vi "DataSimulation.vi"(8 "error in (no error)":errorcluster) -> (0 "error out":errorcluster)   [LabVIEW 2020]
uses:
  StateGPSUpdate.ctl
  <vilib>/Skyline/Message/NI Skyline Message.lvclass
  <vilib>/Skyline/Tag/Shared/typedefs/DataType.ctl
  <vilib>/Skyline/Configuration/Configuration HTTP_class/NI Skyline Configuration HTTP.lvclass/NI Skyline Configuration HTTP.ctl
  TestData.ctl
  <vilib>/Skyline/Configuration/Configuration HTTP_class/Open Configuration HTTP.vi
  <vilib>/Skyline/Message/HTTP Wrapper/NI Skyline Message HTTP.lvclass
  C:/Program Files (x86)/National Instruments/LabVIEW 2020/vi.lib/Skyline/Message/NI Skyline Message.lvclass
  <vilib>/Skyline/Configuration/HTTP/Open Configuration (Desktop).vi
  <vilib>/Skyline/Tag/Wrapper/Wrapper HTTP_class/Open Tag HTTP.vi
  <vilib>/Skyline/Tag/Wrapper/Wrapper_class/Write Tag (Timestamp).vi
  <vilib>/Skyline/Message/HTTP Wrapper/Open (HTTP).vi
  <vilib>/Skyline/Tag/Wrapper/Wrapper_class/Write Tag (Boolean).vi
  <vilib>/Skyline/Configuration/Configuration HTTP_class/NI Skyline Configuration HTTP.lvclass
  <vilib>/Skyline/Configuration/Configuration_class/NI Skyline Configuration.lvclass
  <vilib>/Skyline/Utilities/NI Skyline Utilities.lvlib
  <vilib>/Skyline/Tag/Wrapper/Wrapper_class/NI Skyline Tag.lvclass
  <vilib>/Skyline/Tag/Shared/NI Skyline Tag.lvlib
  <vilib>/Skyline/Tag/Wrapper/Wrapper HTTP_class/NI Skyline Tag HTTP.lvclass
panel:
  in  "stop":bool
  out "Connection Status":bool
  out "SystemStartTime":timestamp
  in  "Test Drive Distance":dbl=1000.0
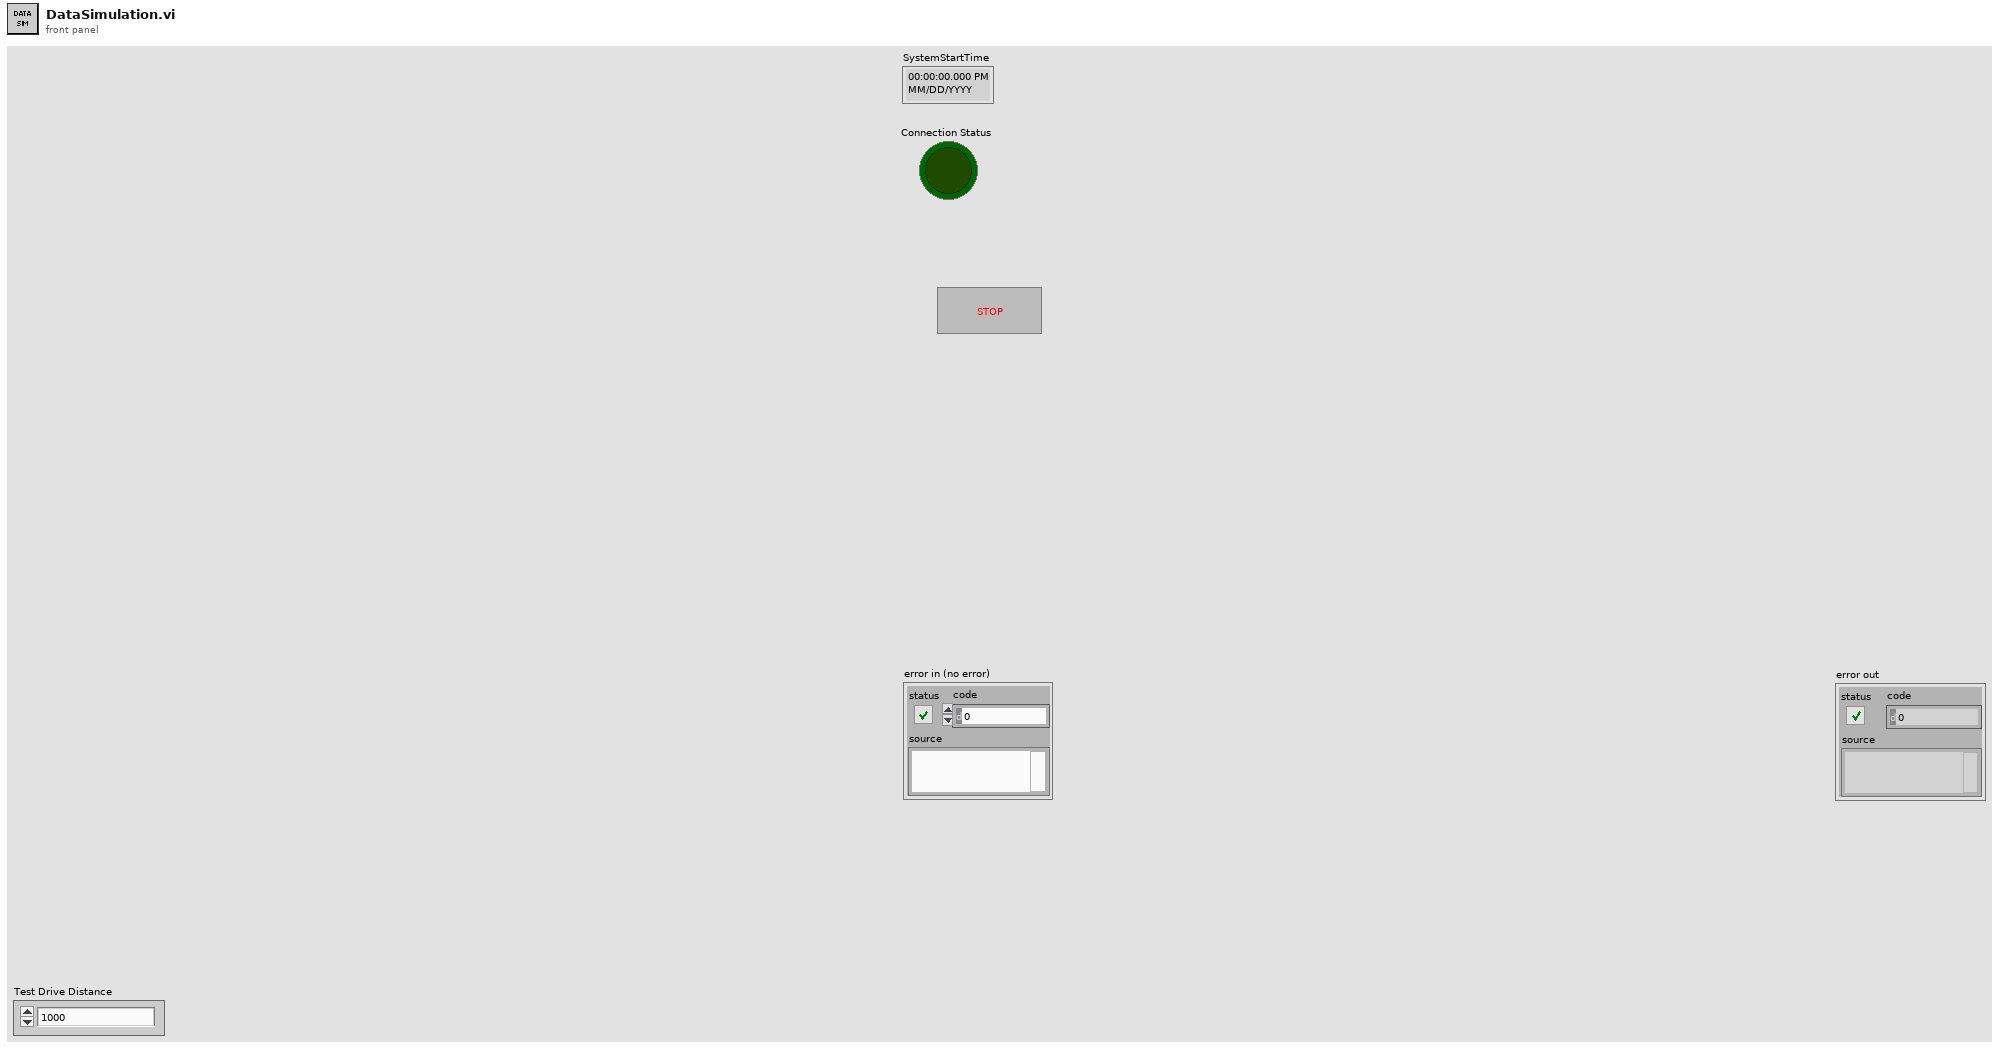
[diagram p1: front panel]
types:
  T1 = typedef "StateGPSUpdate.ctl" = enum16{"Init", "UpdateGPS", "Shutdown"}
  T2 = typedef "NI Skyline Tag.lvlib/DataType.ctl" = enum32{"Double", "I32", "String", "Boolean", "U64", "Timestamp"}
  T3 = typedef "TestData.ctl" = cluster{"GPS":cluster{"Latitude":dbl, "Longitude":dbl, "Timestamp":string}, "SystemLinkClientInfo":cluster{"TargetName":string, "MinionID":string}, "CampaignData":cluster{"DistanceTraveled":dbl, "CampaignProgress":dbl, "Speed":dbl, "Moving":bool}}
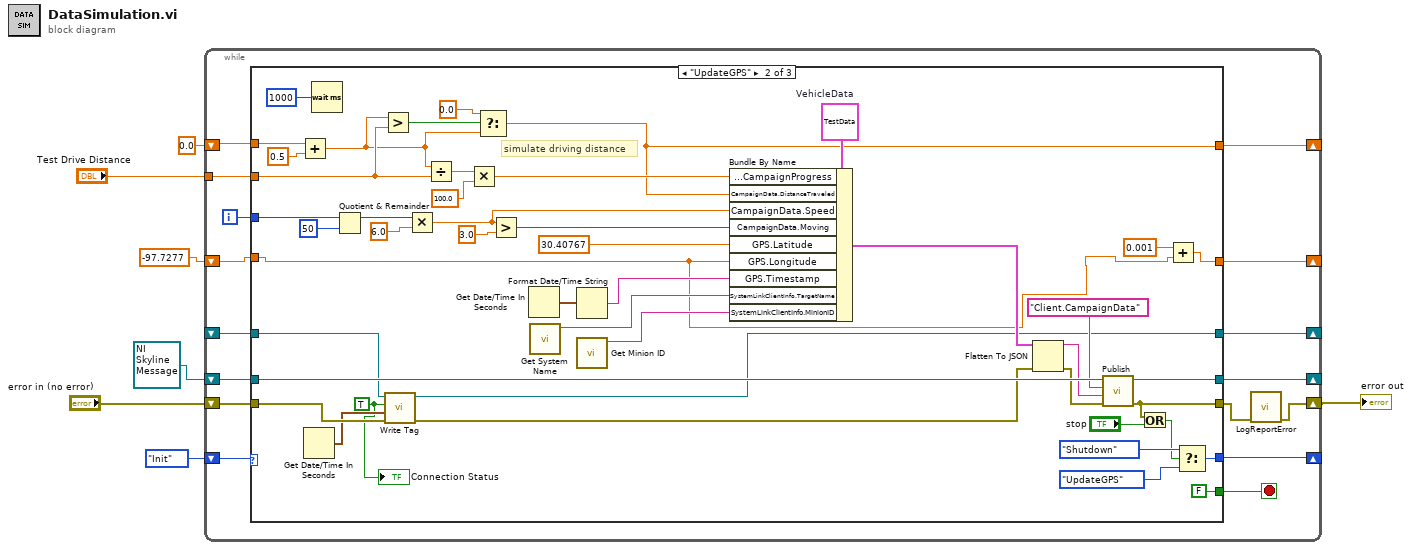
[diagram p0: block diagram]
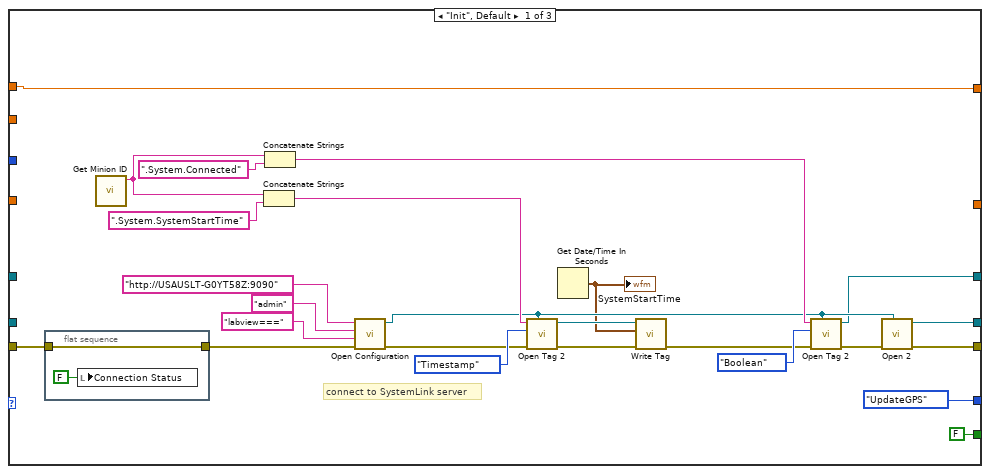
[diagram p2: hidden frame]
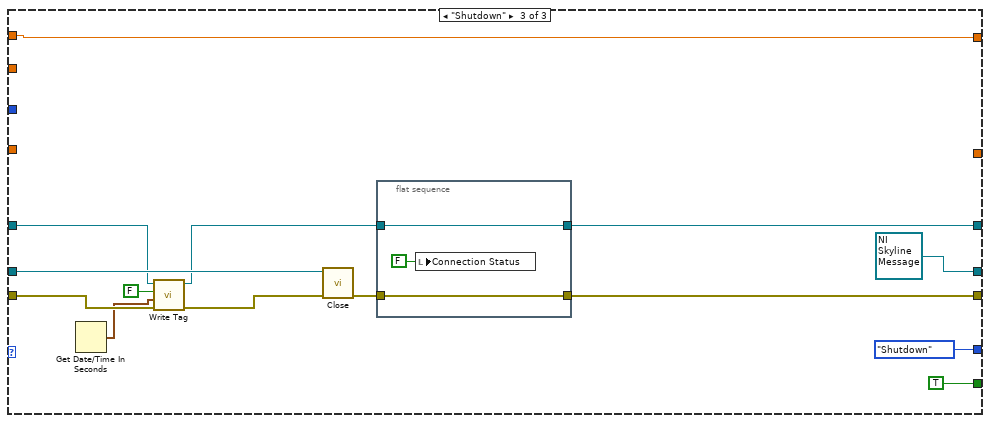
[diagram p3: hidden frame]
diagram:
  n1 = while {
    shift-right: [w12] -> w3
    shift-left: "error in (no error)" -> [w20]
    shift-right: [w21] -> _
    shift-left: StateGPSUpdate."Init" -> [w23]
    shift-right: [w22] -> _
    shift-left: refnum<class "NI Skyline Message.lvclass"> refnum ("message session out") -> [w18]
    tunnel: "Test Drive Distance" -> [w16]
    shift-right: [w15] -> _
    shift-left: 0.0 -> [w14]
    shift-right: [w11] -> _
    shift-left: _ -> [w10]
    shift-right: [w8] -> _
    shift-left: -97.7277 -> [w9]
    i -> [w17]
    stop <- w19 stop-if-true
    n2 = case shown="\"UpdateGPS\"" w23 {
      tunnel: [w45 w96 w103] -> w13
      tunnel: [w44 w90 refnum<class "NI Skyline Message.lvclass"> refnum ("message session out")] -> w22
      tunnel: [StateGPSUpdate."UpdateGPS" w94 StateGPSUpdate."Shutdown"] -> w21
      tunnel: w20 -> [w26 w83 w107]
      tunnel: [FALSE ("stop") FALSE ("stop") TRUE] -> w19
      tunnel: w18 -> [_ w89 w108]
      tunnel: w17 -> [_ w70 _]
      tunnel: w16 -> [_ w65 _]
      tunnel: [w42 w61 w105] -> w15
      tunnel: w14 -> [w42 w74 w105]
      tunnel: [w27 w54 w97] -> w11
      tunnel: w10 -> [_ w59 w101]
      tunnel: w9 -> [_ w52 _]
      tunnel: [_ w53 _] -> w8
      frame "Init", Default {
        # "connect to SystemLink server"
        n3 = flat-sequence {
          tunnel: w26 -> [w49]
          tunnel: [w49] -> w25
          frame #0 {
            n4 = local write "Connection Status"(FALSE ("Connection Status")) -> ()
          }
        }
        n5 = call <vilib>:"Get Minion ID.vi"() -> ("minion id"=w40:string)  [unwired: 11 in]
        n6 = Concatenate Strings(w40, ".System.SystemStartTime" ("path")) -> (w33:string)
        n7 = Concatenate Strings(w40, ".System.Connected" ("path")) -> (w32:string)
        n8 = call-poly <vilib>:"Open Configuration.vi"("error in (no error)"=w25, "password"="labview===", "username"="admin", "server url"="http://USAUSLT-G0YT58Z:9090") -> ("error out"=w36:errorcluster, "configuration"=w31:refnum<class "NI Skyline Configuration HTTP.lvclass">)  [unwired: 6 in]
        n9 = call-poly <vilib>:"Open Tag 2.vi"("configuration"=w31, "error in (no error)"=w36, "Data Type"=DataType."Timestamp", "path"=w33) -> ("error out"=w35:errorcluster, "tag"=w29:refnum<class "NI Skyline Tag.lvclass">)  [unwired: 6 in]
        n10 = Get Date/Time In Seconds() -> (seconds since 1Jan1904=w28:timestamp)
        "SystemStartTime" <- w28
        n11 = call-poly <vilib>:"Write Tag.vi"("error in (no error)"=w35, "value"=w28, "tag in"=w29) -> ("error out"=w30:errorcluster)  [unwired: 7 in, 1 out]
        n12 = call-poly <vilib>:"Open Tag 2.vi"("configuration"=w31, "error in (no error)"=w30, "Data Type"=DataType."Boolean", "path"=w32) -> ("error out"=w34:errorcluster, "tag"=w27:refnum<class "NI Skyline Tag.lvclass">)  [unwired: 6 in]
        n13 = call-poly <vilib>:"Open 2.vi"("configuration"=w31, "error in (no error)"=w34) -> ("error out"=w45:errorcluster, "message session"=w44:refnum<class "NI Skyline Message HTTP.lvclass">)  [unwired: 8 in]
      }
      frame "UpdateGPS" {
        w57 = TRUE ("value")
        w88 = T3 {"GPS"={"Latitude"=0.0, "Longitude"=0.0, "Timestamp"=""}, "SystemLinkClientInfo"={"TargetName"="", "MinionID"=""}, "CampaignData"={"DistanceTraveled"=0.0, "CampaignProgress"=0.0, "Speed"=0.0, "Moving"=FALSE}}  # VehicleData
        # "simulate driving distance"
        n14 = Add(x=w74, y=0.5) -> (x+y=w63:dbl)
        n15 = Get Date/Time In Seconds() -> (seconds since 1Jan1904=w58:timestamp)
        n16 = Wait (ms)(milliseconds to wait=u32 1000) -> ()  [unwired: 1 out]
        n17 = Quotient & Remainder(x=w70, y=50) -> (x-y*floor(x/y)=w67:i32)  [unwired: 1 out]
        n18 = Greater?(x=w63, y=w65) -> (0:w64:bool)
        n19 = call-poly <vilib>:"Write Tag.vi"("error in (no error)"=w83, "time stamp"=w58, "value"=w57, "tag in"=w59) -> ("error out"=w60:errorcluster, "tag out"=w54:refnum<class "NI Skyline Tag.lvclass">)  [unwired: 6 in]
        n20 = Multiply(x=w67, y=6.0) -> (x*y=w66:dbl)
        n21 = Divide(x=w63, y=w65) -> (x/y=w77:dbl)
        n22 = Multiply(x=w77, y=100.0) -> (x*y=w75:dbl)
        n23 = Select(t=0.0, s=w64, f=w63) -> (s? t:f=w61:dbl)
        n24 = Greater?(x=w66, y=3.0) -> (0:w72:bool)
        n25 = Get Date/Time In Seconds() -> (seconds since 1Jan1904=w86:timestamp)
        n26 = call <vilib>:"Get System Name.vi"() -> ("system name"=w80:string)  [unwired: 11 in]
        n27 = Format Date/Time String(seconds (now)=w86) -> (date/time string=w85:string)  [unwired: 2 in]
        n28 = call <vilib>:"Get Minion ID.vi"() -> ("minion id"=w79:string)  [unwired: 11 in]
        n29 = Bundle By Name(cluster=w88, "CampaignData.CampaignProgress"=w75, "CampaignData.DistanceTraveled"=w61, "CampaignData.Speed"=w66, "CampaignData.Moving"=w72, "GPS.Latitude"=30.40767, "GPS.Longitude"=w52, "GPS.Timestamp"=w85, "SystemLinkClientInfo.TargetName"=w80, "SystemLinkClientInfo.MinionID"=w79) -> (w84:T3)
        n30 = Flatten To JSON(anything=w84, error in (no error)=w60) -> (JSON string=w87:string, 11:w82:errorcluster)  [unwired: 1 in]
        n31 = call-dynamic "Publish.vi"("error in (no error)"=w82, "message"=w87, "topic"="Client.CampaignData", "message session in"=w89) -> ("error out"=w96:errorcluster, "message session out"=w90:refnum<class "NI Skyline Message.lvclass">)  [unwired: 6 in]
        n32 = Or(x=w96, y="stop") -> (x .or. y?=w91:bool)
        n33 = Add(x=0.001, y=w52) -> (x+y=w53:dbl)
        n34 = Select(t=StateGPSUpdate."Shutdown", s=w91, f=StateGPSUpdate."UpdateGPS") -> (s? t:f=w94:T1)
        "Connection Status" <- w57
      }
      frame "Shutdown" {
        n35 = Get Date/Time In Seconds() -> (seconds since 1Jan1904=w99:timestamp)
        n36 = call-poly <vilib>:"Write Tag.vi"("error in (no error)"=w107, "time stamp"=w99, "value"=FALSE, "tag in"=w101) -> ("error out"=w102:errorcluster, "tag out"=w98:refnum<class "NI Skyline Tag.lvclass">)  [unwired: 6 in]
        n37 = call-dynamic "Close.vi"("error in (no error)"=w102, "message session"=w108) -> ("error out"=w104:errorcluster)  [unwired: 9 in]
        n38 = flat-sequence {
          tunnel: w104 -> [w112]
          tunnel: [w112] -> w103
          tunnel: w98 -> [w111]
          tunnel: [w111] -> w97
          frame #0 {
            n39 = local write "Connection Status"(FALSE ("Connection Status")) -> ()
          }
        }
      }
    }
    n40 = call "LogReportError.vi"("error in (no error)"=w13) -> ("error out"=w12:errorcluster)  [unwired: 10 in]
  }
  "error out" <- w3
